vi "Shared_Variable_test_2.vi"() -> ()   [LabVIEW 2016]
panel:
  out "Reading current time":timestamp
  in  "Stop Button":bool
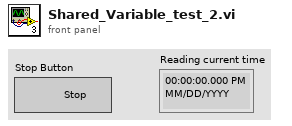
[diagram p1: front panel]
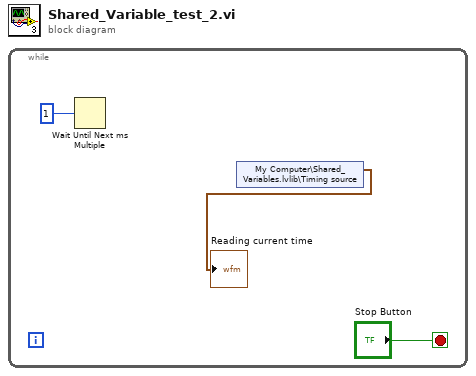
[diagram p0: block diagram]
diagram:
  n1 = while {
    stop <- "Stop Button" stop-if-true
    n2 = Wait Until Next ms Multiple(millisecond multiple=u32 1) -> ()  [unwired: 1 out]
    n3 = shared-variable "My Computer\\Shared_Variables.lvlib\\Timing source"() -> (→"Reading current time":timestamp)  [unwired: 1 in, 1 out]
  }
